vi "Table - Colour Single Row.vi"(5 "Highlight":u32(colorbox)=8108276, 6 "Clear Table? (T)":bool=TRUE, 7 "Default":u32(colorbox)=16448250, 8 "error in (no error)":errorcluster, 10 "Row To Colour":i32, 11 "Table To Colour":refnum<vi>) -> (0 "error out":errorcluster)   [LabVIEW 2015, in "Utility.lvlib"]
doc: "Colours a single row of a table with the <b>Highlight</b> colour.\n\nThis VI optionally clears all colouring from the table (by colouring all rows with the Default colour first) if the the <b>Clear Table?</b> input is set. This is the default action.\n\nTwo special modes of operation for this VI exist:\n if <b>Row To Colour</b> is -2 then all the rows will be coloured with the <b>Highlight</b> colour\n if <b>Row To Colour</b> is <= -3 then the row colouring is disabled (this is useful to perform only the clearing of the colouring)"
uses:
  Utility.lvlib
  <vilib>/Utility/miscctls.llb/LVRowAndColumnTypeDef.ctl
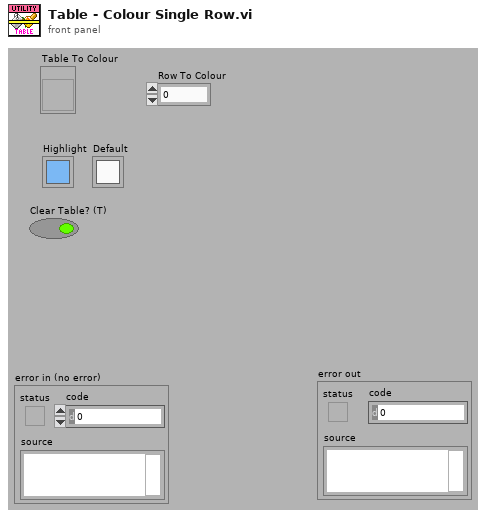
[diagram p1: front panel]
types:
  T1 = typedef "LVRowAndColumnTypeDef.ctl" = cluster{"Row":i32, "Column":i32}
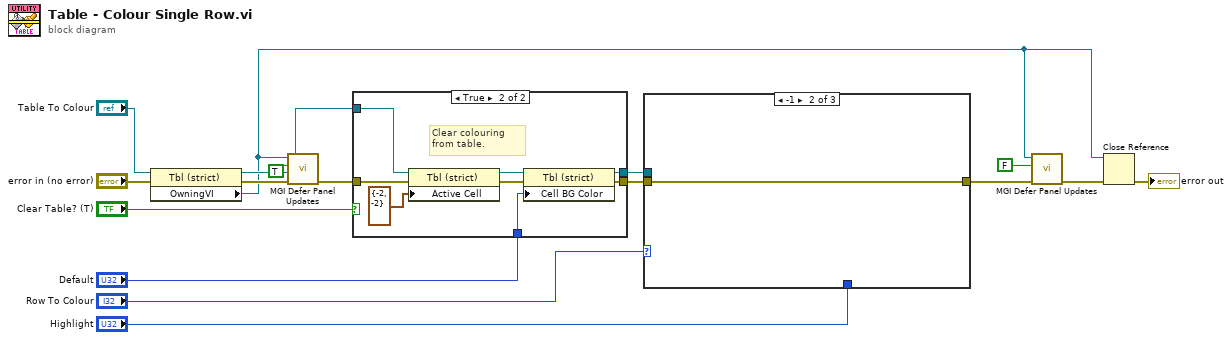
[diagram p0: block diagram]
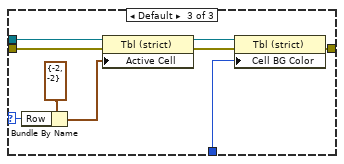
[diagram p3: hidden frame]
diagram:
  n1 = property class="Tbl (strict)"(reference="Table To Colour", error in="error in (no error)") -> (reference out=w6:refnum<vi>, error out=w4:errorcluster, "OwningVI"=w1:refnum<vi>)
  n2 = call <userlib>:"MGI Defer Panel Updates.vi"("Error In"=w4, "Defer Updates?"=TRUE ("Defer Updates? (False: Restore state)"), "VI Reference (Caller)"=w1) -> ("Error Out"=w13:errorcluster)  [unwired: 8 in]
  n3 = case shown="True" "Clear Table? (T)" {
    tunnel: w6 -> [w19 w27]
    tunnel: "Default" -> [_ w24]
    tunnel: [w19 w23] -> w16
    tunnel: [w18 w22] -> w15
    tunnel: w13 -> [w18 w21]
    frame False {
    }
    frame True {
      # "Clear colouring from table."
      n4 = property class="Tbl (strict)"(reference=w27, error in=w21, "Active Cell"=T1 {"Row"=-2, "Column"=-2} ("Active Cell:Active Cell")) -> (reference out=w26:refnum<vi>, error out=w25:errorcluster)
      n5 = property class="Tbl (strict)"(reference=w26, error in=w25, "Cell BG Color"=w24) -> (reference out=w23:refnum<vi>, error out=w22:errorcluster)
    }
  }
  n6 = case shown="-1" "Row To Colour" {
    selector: "Row To Colour" -> [_ _ w30]
    tunnel: w16 -> [_ _ w38]
    tunnel: w15 -> [w28 w29 w35]
    tunnel: "Highlight" -> [_ _ w32]
    tunnel: [w28 w29 w31] -> w12
    frame ..-3 {
    }
    frame -1 {
    }
    frame Default {
      n7 = Bundle By Name(cluster=T1 {"Row"=-2, "Column"=-2} ("Active Cell:Active Cell"), "Row"=w30) -> (w36:T1)
      n8 = property class="Tbl (strict)"(reference=w38, error in=w35, "Active Cell"=w36) -> (reference out=w34:refnum<vi>, error out=w33:errorcluster)
      n9 = property class="Tbl (strict)"(reference=w34, error in=w33, "Cell BG Color"=w32) -> (error out=w31:errorcluster)  [unwired: 1 out]
    }
  }
  n10 = call <userlib>:"MGI Defer Panel Updates.vi"("Error In"=w12, "Defer Updates?"=FALSE ("Defer Updates? (False: Restore state)"), "VI Reference (Caller)"=w1) -> ("Error Out"=w3:errorcluster)  [unwired: 1 in, 7 out]
  n11 = Close Reference(reference=w1, error in (no error)=w3) -> (error out=→"error out":errorcluster)
